vi "Shooting Motor Start Stop.vi"(10 "Stop":bool, 11 "Start":bool) -> (2 "Ready To Shoot":bool=TRUE)   [LabVIEW 2012]
panel:
  in  "Time to Spin Up (ms)":dbl=1000.0
  in  "Speed":dbl=1.0
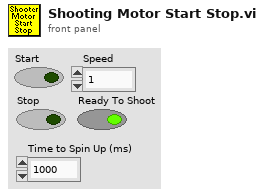
[diagram p1: front panel]
types:
  T1 = typedef "WPI_MotorControlDeviceRef.ctl" = cluster{"DeviceStatus":errorcluster, "Type":enum16{"PWM", "CAN"}, "PWM":cluster{"Digital Module":T2, "PWM Channel":T3, "DeadBand":T4}, "CAN":cluster{"Device Number":u8, "Control Mode":T5, "Semaphore":T6, "Max Vout":dbl}, "Invert":bool, "TransformRef":T7, "InvTransformRef":T7}
  T2 = typedef "FPGA_TypedefDigitalModule.ctl" = enum16{"Digital Module 1", "Digital Module 2"}
  T3 = typedef "FPGA_DIOPWMChannel.ctl" = enum8{"PWM 1", "PWM 2", "PWM 3", "PWM 4", "PWM 5", "PWM 6", "PWM 7", "PWM 8", "PWM 9", "PWM 10", "Invalid"}
  T4 = typedef "WPI_PWMDeadband.ctl" = cluster{"Name":string, "maxPositivePwm":i32, "minPositivePwm":i32, "centerPwm":i32, "maxNegativePwm":i32, "minNegativePwm":i32, "angularRange":u16}
  T5 = typedef "WPI_CANJaguar_ControlMode.ctl" = enum8{"Percent VBus", "Current", "Speed", "Position", "Voltage"}
  T6 = typedef "Semaphore RefNum" = refnum<k1>
  T7 = typedef "WPI_PWMTransform_ConPane.ctl" = refnum<vi>
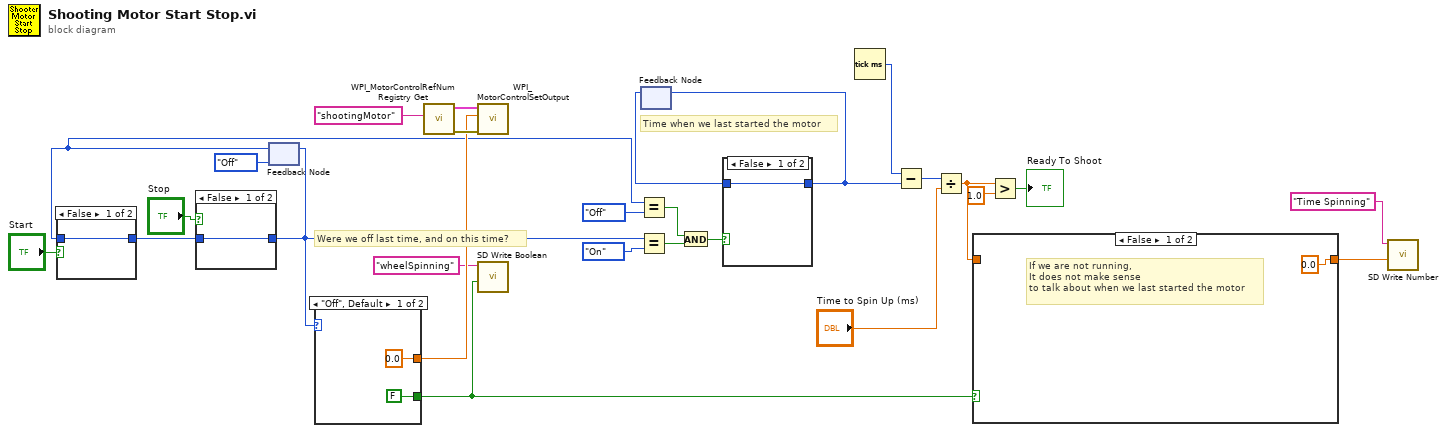
[diagram p0: block diagram]
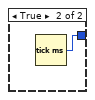
[diagram p3: hidden frame]
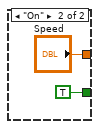
[diagram p4: hidden frame]
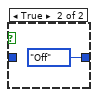
[diagram p5: hidden frame]
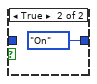
[diagram p6: hidden frame]
diagram:
  # "Time when we last started the motor"
  # "Were we off last time, and on this time?"
  n1 = feedback #1(enum16{"Off", "On"}."Off") -> (w19:enum16{"Off", "On"})
  n2 = case shown="False" "Start" {
    tunnel: w19 -> [w28 _]
    tunnel: [w28 enum16{"Off", "On"}."On"] -> w23
    frame False {
    }
    frame True {
    }
  }
  n3 = case shown="False" "Stop" {
    tunnel: [w30 enum16{"Off", "On"}."Off"] -> w17
    tunnel: w23 -> [w30 _]
    frame False {
    }
    frame True {
    }
  }
  n4 = feedback-in #1(w17) -> ()
  n5 = case shown="\"Off\", Default" w17 {
    tunnel: [0.0 ("Speed") "Speed"] -> w20
    tunnel: [FALSE TRUE] -> w4
    frame "Off", Default {
    }
    frame "On" {
    }
  }
  n6 = call <vilib>:"WPI_MotorControlRefNum Registry Get.vi"("refnum name"="shootingMotor") -> ("error out"=w22:errorcluster, "MotorControlDevRef"=w21:T1)  [unwired: 9 in]
  n7 = call <vilib>:"WPI_MotorControlSetOutput.vi"("error in (no error)"=w22, "Output"=w20, "MotorControlDevRef"=w21) -> ()  [unwired: 6 in, 3 out]
  n8 = call <vilib>:"SD Write Boolean.vi"("Boolean"=w4, "Name"="wheelSpinning") -> ()  [unwired: 8 in, 2 out]
  n9 = Equal?(x=w19, y=enum16{"Off", "On"}."Off") -> (x = y?=w14:bool)
  n10 = Equal?(x=w17, y=enum16{"Off", "On"}."On") -> (x = y?=w15:bool)
  n11 = feedback #2() -> (w12:u32)  [unwired: 1 in]
  n12 = And(x=w14, y=w15) -> (x .and. y?=w13:bool)
  n13 = case shown="False" w13 {
    tunnel: [w36 w37] -> w10
    tunnel: w12 -> [w36 _]
    frame False {
    }
    frame True {
      n14 = Tick Count (ms)() -> (millisecond timer value=w37:u32)
    }
  }
  n15 = feedback-in #2(w10) -> ()
  n16 = Tick Count (ms)() -> (millisecond timer value=w11:u32)
  n17 = Subtract(x=w11, y=w10) -> (x-y=w9:u32)
  n18 = Divide(x=w9, y="Time to Spin Up (ms)") -> (x/y=w3:dbl)
  n19 = case shown="False" w4 {
    tunnel: w3 -> [_ w39]
    tunnel: [0.0 w39] -> w6
    frame False {
      # "If we are not running,\nIt does not make sense\nto talk about when we last started the motor"
    }
    frame True {
    }
  }
  n20 = Greater?(x=w3, y=1.0) -> (0:→"Ready To Shoot":bool)
  n21 = call <vilib>:"SD Write Number.vi"("Numeric"=w6, "Name"="Time Spinning") -> ()  [unwired: 8 in, 2 out]
